vi "RL-Spect-Fast.vi"   [LabVIEW 2014]
doc: "Random Laser Project\n\nAndré Romero - 2020\nandretec@ifsc.usp.br\n\nMain Program"
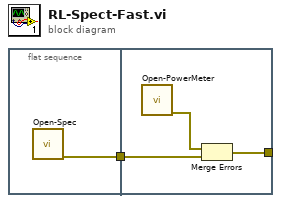
[diagram p0: block diagram]
diagram:
  n1 = flat-sequence {
    tunnel: [w2] -> w1
    tunnel: w1 -> [w4]
    tunnel: [w3] -> _
    frame #0 {
      n2 = call "Open-Spec.vi"() -> ("error out"=w2:errorcluster)  [unwired: 9 in, 2 out]
    }
    frame #1 {
      n3 = call "Open-PowerMeter.vi"() -> ("error out"=w5:errorcluster)  [unwired: 10 in, 1 out]
      n4 = Merge Errors(w5, w4) -> (w3:errorcluster)
    }
  }
